vi "波形图表的多图线布置方式.vi"() -> ()   [LabVIEW 2010]
uses:
  <vilib>/Analysis/NI_AALBase.lvlib
panel:
  out "波形图表 2":cluster{dbl, dbl}[](graph)
  out "波形图表":cluster{dbl, dbl}[](graph)
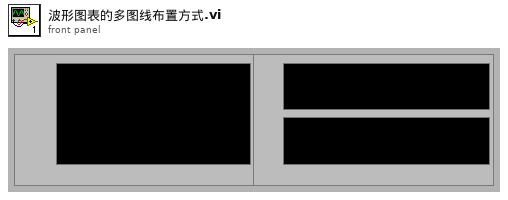
[diagram p1: front panel]
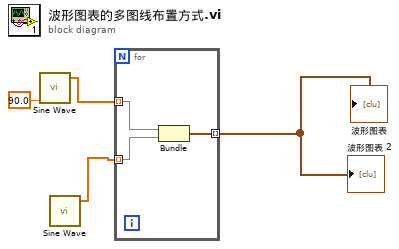
[diagram p0: block diagram]
diagram:
  n1 = call <vilib>:"Sine Wave.vi"("phase in"=90.0) -> ("sine wave"=w3:dbl[])  [unwired: 4 in, 2 out]
  n2 = call <vilib>:"Sine Wave.vi"() -> ("sine wave"=w2:dbl[])  [unwired: 5 in, 2 out]
  n3 = for {
    tunnel: w3 -> [w7] mode=indexing
    tunnel: w2 -> [w6] mode=indexing
    tunnel: [w5] -> w1 mode=indexing
    n4 = Bundle(w7, w6) -> (w5:cluster{dbl, dbl})  [unwired: 1 in]
  }
  "波形图表" <- w1
  "波形图表 2" <- w1
